vi "Case_Numerico.vi"() -> ()   [LabVIEW 2016]
panel:
  in  "Ring":u16(ring) items=["Resta", "Suma", "Multiplicacion", "División"]
  out "Numeric Indicator":dbl
  in  "B":dbl
  in  "A":dbl
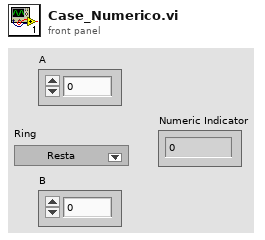
[diagram p1: front panel]
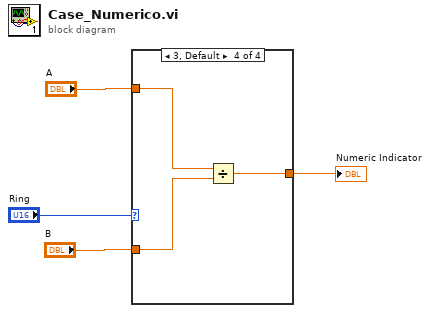
[diagram p0: block diagram]
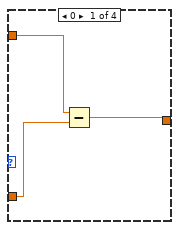
[diagram p2: hidden frame]
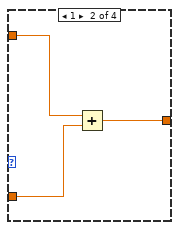
[diagram p3: hidden frame]
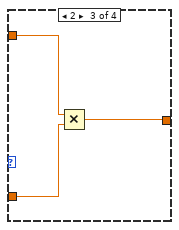
[diagram p4: hidden frame]
diagram:
  n1 = case shown="3, Default" "Ring" {
    tunnel: "A" -> [w6 w10 w13 w14]
    tunnel: "B" -> [w5 w9 w12 w16]
    tunnel: [w7 w8 w11 w15] -> w2
    frame 0 {
      n2 = Subtract(x=w6, y=w5) -> (x-y=w7:dbl)
    }
    frame 1 {
      n3 = Add(x=w10, y=w9) -> (x+y=w8:dbl)
    }
    frame 2 {
      n4 = Multiply(x=w13, y=w12) -> (x*y=w11:dbl)
    }
    frame 3, Default {
      n5 = Divide(x=w14, y=w16) -> (x/y=w15:dbl)
    }
  }
  "Numeric Indicator" <- w2
